vi "DAQmx Creation.vi"() -> ()   [LabVIEW 2019]
uses:
  <vilib>/DAQmx/read.llb/DAQmx Read (Analog DBL 1Chan 1Samp).vi
  <vilib>/DAQmx/miscellaneous.llb/DAQmx Fill In Error Info.vi
panel:
  out "System current state":string
  out "Threshold exceeded":bool=TRUE
  in  "Maximum Temperature (Deg C)":dbl format="%0.2f"
  out "error out":errorcluster
  out "Current Temperature (deg C)":dbl format="%0.2f"
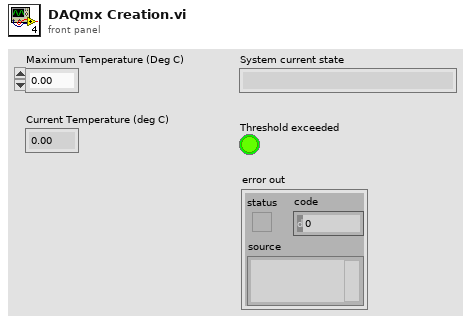
[diagram p1: front panel]
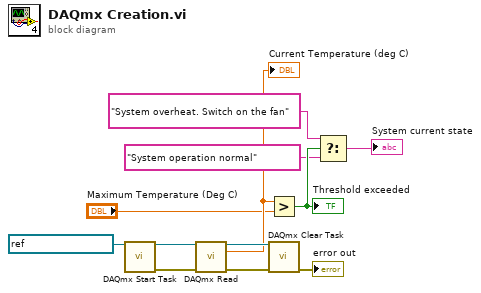
[diagram p0: block diagram]
diagram:
  n1 = call <vilib>:"DAQmx Start Task.vi"("task/channels in"=refnum<k21> "Thermocouple" ("task out")) -> ("task out"=w8:refnum<k21>, "error out"=w11:errorcluster)  [unwired: 13 in]
  n2 = call-poly <vilib>:"DAQmx Read.vi"("task/channels in"=w8, "error in"=w11) -> ("task out"=w7:refnum<k21>, "data"=w6:dbl, "error out"=w10:errorcluster)  [unwired: 11 in]
  "Current Temperature (deg C)" <- w6
  n3 = Greater?(x=w6, y="Maximum Temperature (Deg C)") -> (0:w4:bool)
  "Threshold exceeded" <- w4
  n4 = call <vilib>:"DAQmx Clear Task.vi"("task in"=w7, "error in"=w10) -> ("error out"=→"error out":errorcluster)  [unwired: 13 in]
  n5 = Select(t="System overheat. Switch on the fan", s=w4, f="System operation normal") -> (s? t:f=→"System current state":string)
